vi "LabVIEW Type to JSON Tree Generator.vi"(8 "error in (no error)":errorcluster, 11 "Cluster":T1={"Zip Code"=78758, "Name"="National Instruments", "Is Awesome?"=TRUE, "Products"=[]}) -> (0 "error out":errorcluster, 3 "JSON Tree Passthrough":variant)   [LabVIEW 2011]
uses:
  LabVIEW Type to JSON Tree Data.ctl
  i3-json.lvlib
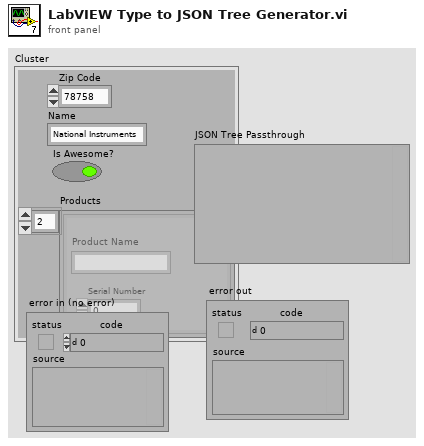
[diagram p1: front panel]
types:
  T1 = typedef "LabVIEW Type to JSON Tree Data.ctl" = cluster{"Zip Code":i32, "Name":string, "Is Awesome?":bool, "Products":cluster{"Product Name":string, "Serial Number":u32}[]}
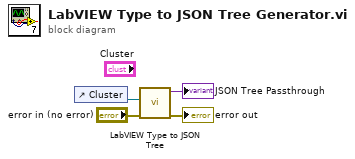
[diagram p0: block diagram]
diagram:
  n1 = control-ref of="Cluster"() -> (w2:refnum<vi>)
  n2 = call "LabVIEW Type to JSON Tree.vi"("error in (no error)"="error in (no error)", "Ctl Refnum"=w2) -> ("error out"=→"error out":errorcluster, "JSON Tree Out"=→"JSON Tree Passthrough":variant)  [unwired: 8 in]
